vi "RotateStage.vi"(4 "Acceleration":dbl, 5 "Enum":enum16{"PI", "Steinmeyer"}(ring), 6 "Velocity":dbl, 7 "Direction":bool, 8 "Stage max rotation":dbl=365.0, 9 "Stage position":dbl, 10 "Stage step size (deg)":dbl, 11 "PIAxisID":string[](array[string])) -> ()   [LabVIEW 2013]
doc: "This VI rotates the stage with a step in a specified direction.\n\nInputs:\nStage (enum): Specify which stage to rotate. PI or Steinmeyer\nDirection (bool): False for clockwise rotation, true for counterclockwise rotation\nAxisID (array of int): Value for the axisID of the connected stage."
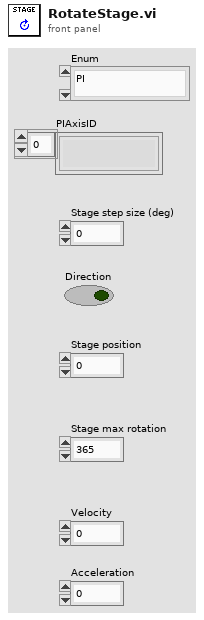
[diagram p1: front panel]
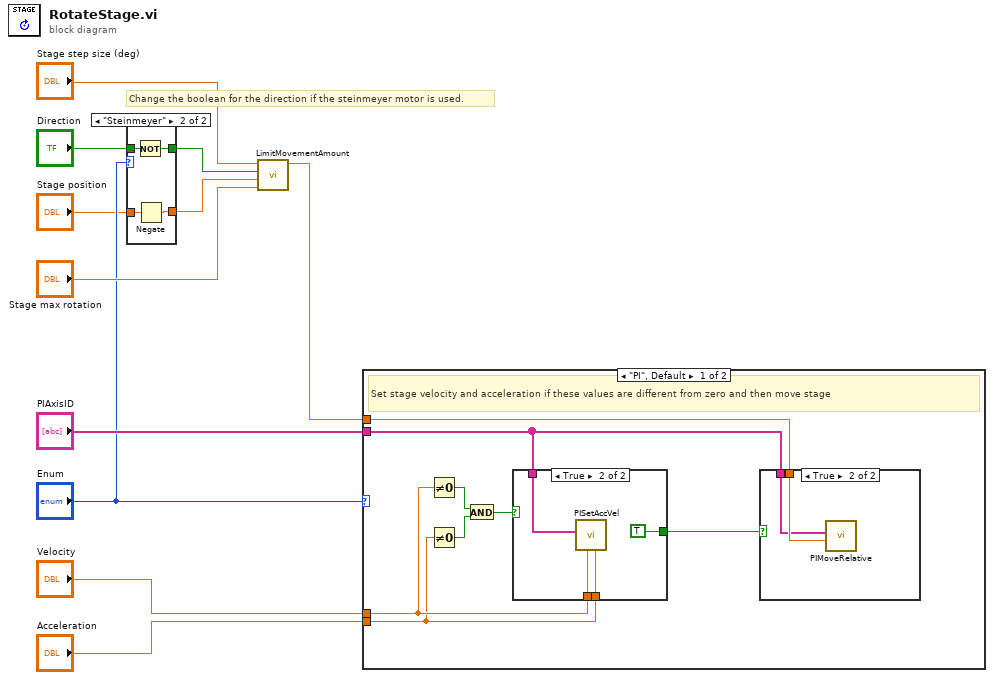
[diagram p0: block diagram]
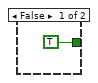
[diagram p4: hidden frame]
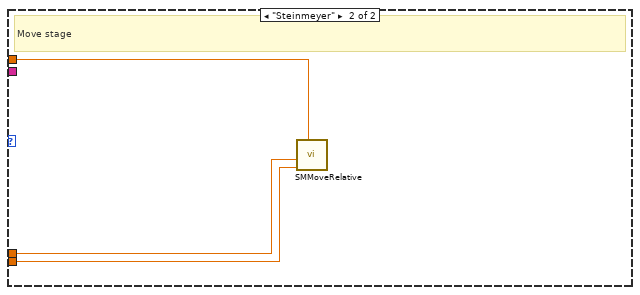
[diagram p5: hidden frame]
diagram:
  # "Change the boolean for the direction if the steinmeyer motor is used."
  n1 = case shown="\"Steinmeyer\"" "Enum" {
    tunnel: "Direction" -> [w13 w16]
    tunnel: [w13 w17] -> w3
    tunnel: "Stage position" -> [w12 w15]
    tunnel: [w12 w14] -> w1
    frame "PI", Default {
    }
    frame "Steinmeyer" {
      n2 = Not(x=w16) -> (.not. x?=w17:bool)
      n3 = Negate(x=w15) -> (-x=w14:dbl)
    }
  }
  n4 = call "LimitMovementAmount.vi"("Max rotation"="Stage max rotation", "Current position"=w1, "Direction"=w3, "Move amount in"="Stage step size (deg)") -> ("Move amount out"=w7:dbl)  [unwired: 6 in, 1 out]
  n5 = case shown="\"PI\", Default" "Enum" {
    tunnel: "Velocity" -> [w22 w35]
    tunnel: "Acceleration" -> [w18 w34]
    tunnel: w7 -> [w20 w33]
    tunnel: "PIAxisID" -> [w19 _]
    frame "PI", Default {
      # "Set stage velocity and acceleration if these values are different from zero and then move stage"
      n6 = Not Equal To 0?(x=w22) -> (x != 0?=w24:bool)
      n7 = Not Equal To 0?(x=w18) -> (x != 0?=w25:bool)
      n8 = And(x=w24, y=w25) -> (x .and. y?=w23:bool)
      n9 = case shown="True" w23 {
        tunnel: w18 -> [_ w32]
        tunnel: w22 -> [_ w31]
        tunnel: [TRUE TRUE] -> w21
        tunnel: w19 -> [_ w29]
        frame False {
        }
        frame True {
          n10 = call "PISetAccVel.vi"("Acceleration"=w32, "Velocity"=w31, "AxisID"=w29) -> ()  [unwired: 8 in, 1 out]
        }
      }
      n11 = case shown="True" w21 {
        tunnel: w20 -> [_ w27]
        tunnel: w19 -> [_ w26]
        frame False {
        }
        frame True {
          n12 = call "PIMoveRelative.vi"("Amount"=w27, "AxisID"=w26) -> ()  [unwired: 9 in, 1 out]
        }
      }
    }
    frame "Steinmeyer" {
      # "Move stage"
      n13 = call "SMMoveRelative.vi"("Displacement"=w33, "Acceleration"=w34, "Speed"=w35) -> ()  [unwired: 8 in, 1 out]
    }
  }
